vi "Caller DVR.vi"(0 "DVR In":refnum<data-value>, 5 "Sub Panel":refnum<vi>, 11 "Error In":errorcluster) -> (4 "DVR Out":refnum<data-value>, 15 "Error Out":errorcluster)   [LabVIEW 2023, in "Arithemetic Operation.lvclass"]
doc: "The method acts as a wrapper to the over riding caller method to call the UI in the sub panel asynchronously."
uses:
  Arithemetic Operation.lvclass
  Typedef/User Event Operations.ctl
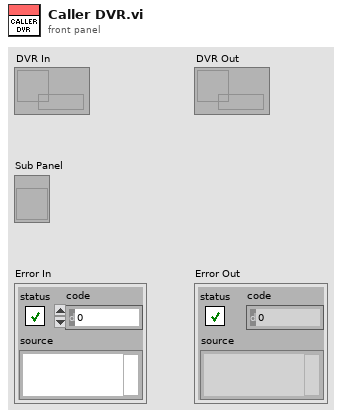
[diagram p1: front panel]
types:
  T1 = typedef "User Event Operations.ctl" = enum16{"Obtain", "Generate", "Release"}
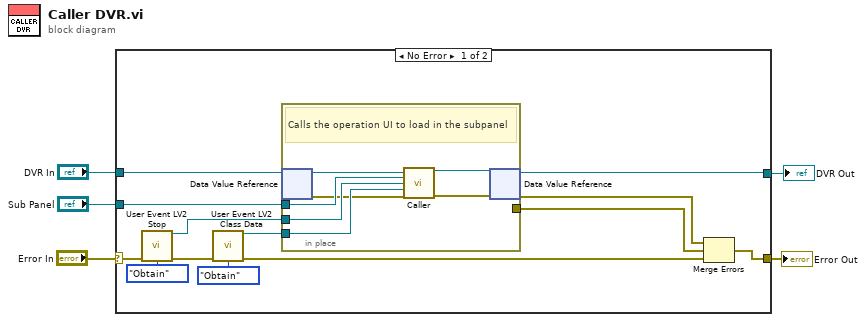
[diagram p0: block diagram]
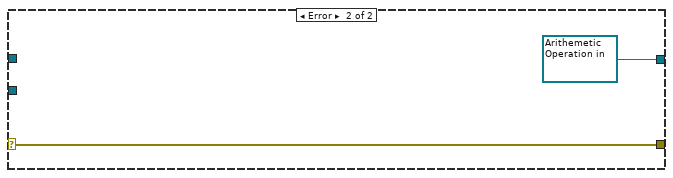
[diagram p2: hidden frame]
diagram:
  n1 = case shown="No Error" "Error In" {
    selector: "Error In" -> [w18 w27]
    tunnel: [w6 w27] -> w4
    tunnel: [w16 refnum<data-value> refnum ("Input")] -> w2
    tunnel: "DVR In" -> [w17 _]
    tunnel: "Sub Panel" -> [w15 _]
    frame No Error {
      n2 = call "User Event LV2 Stop.vi"("Error In"=w18, "Operation"=User_Event_Operations."Obtain") -> ("User Event Ref"=w10:refnum<user-event>, "Error Out"=w12:errorcluster)  [unwired: 12 in]
      n3 = call "User Event LV2 Class Data.vi"("Error In"=w12, "Operation"=User_Event_Operations."Obtain") -> ("User Event Ref"=w14:refnum<user-event>, "Error Out"=w7:errorcluster)  [unwired: 12 in]
      n4 = in-place {
        in-place-border: w15 -> [w23]
        in-place-border: w10 -> [w22]
        in-place-border: w14 -> [w21]
        in-place-border: [w19] -> w8
        # "Calls the operation UI to load in the subpanel"
        n5 = in-place-dvr #1(w17) -> (w25:refnum<class "Arithemetic Operation.lvclass">, w20:errorcluster)
        n6 = call-dynamic "Caller.vi"("Arithemetic Operation in"=w25, "Sub Panel"=w23, "State"=w22, "Class Data"=w21, "Error In"=w20) -> ("Arithemetic Operation out"=w24:refnum<class "Arithemetic Operation.lvclass">, "Error Out"=w19:errorcluster)  [unwired: 9 in]
        n7 = in-place-dvr #1(w24) -> (w16:refnum<data-value>, w9:errorcluster)
      }
      n8 = Merge Errors(w9, w8, w7) -> (w6:errorcluster)
    }
    frame Error {
    }
  }
  "Error Out" <- w4
  "DVR Out" <- w2
